vi "USB6343_Control_v1.6.2.vi"(8 "error in":errorcluster caption="错误输出", 10 "interface":T2, 11 "tasks":T3) -> ()   [LabVIEW 2013]
uses:
  <vilib>/DAQmx/read.llb/DAQmx Read (Analog 1D DBL NChan 1Samp).vi
  <vilib>/DAQmx/read.llb/DAQmx Read (Digital 1D Bool NChan 1Samp 1Line).vi
  <vilib>/DAQmx/read.llb/DAQmx Read (Counter DBL 1Chan 1Samp).vi
  <vilib>/DAQmx/write.llb/DAQmx Write (Digital 1D Bool NChan 1Samp 1Line).vi
  <vilib>/DAQmx/write.llb/DAQmx Write (Analog 1D DBL NChan 1Samp).vi
  <vilib>/DAQmx/miscellaneous.llb/DAQmx Fill In Error Info.vi
  <vilib>/DAQmx/configure/timing.llb/DAQmx Timing (Implicit).vi
panel:
  in  "stop":bool=TRUE
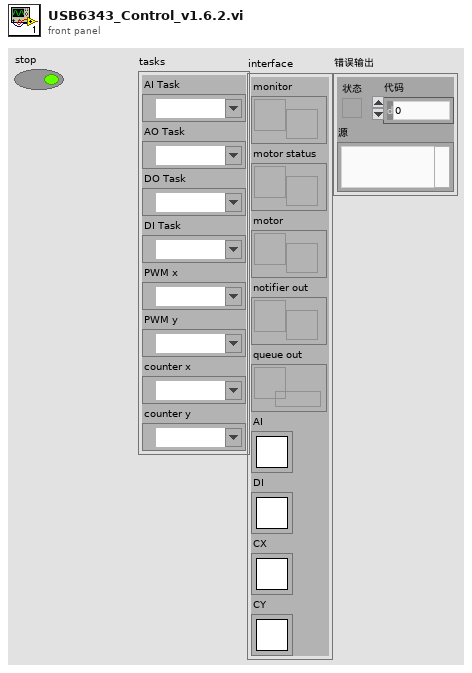
[diagram p1: front panel]
types:
  T1 = typedef "Semaphore RefNum" = refnum<k1>
  T2 = cluster{"monitor":refnum<user-event>, "motor status":refnum<user-event>, "motor":refnum<user-event>, "notifier out":refnum<notifier>, "queue out":refnum<queue>, "AI":T1, "DI":T1, "CX":T1, "CY":T1}
  T3 = cluster{"AI Task":refnum<k21>, "AO Task":refnum<k21>, "DO Task":refnum<k21>, "DI Task":refnum<k21>, "PWM x":refnum<k21>, "PWM y":refnum<k21>, "counter x":refnum<k21>, "counter y":refnum<k21>}
  T4 = cluster{"cmd":string, "channel":i32, "value":dbl, "on/off":bool, "return value":refnum<vi>}
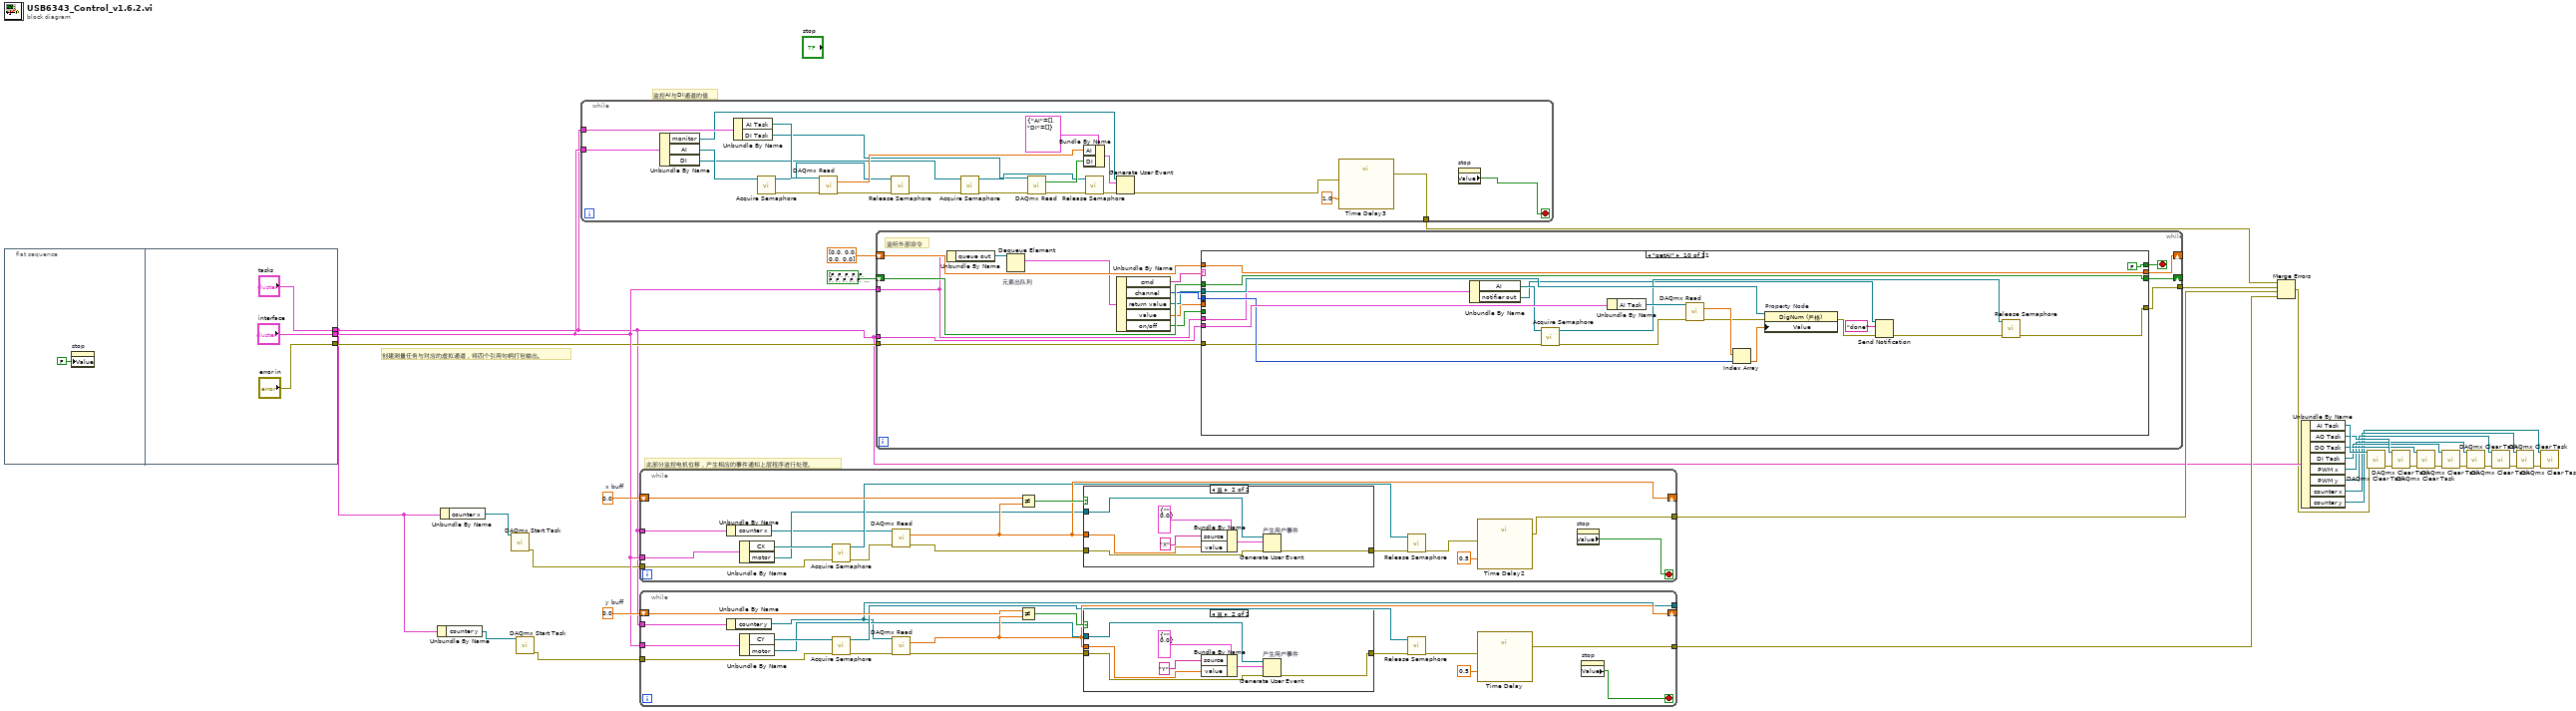
[diagram p0: block diagram]
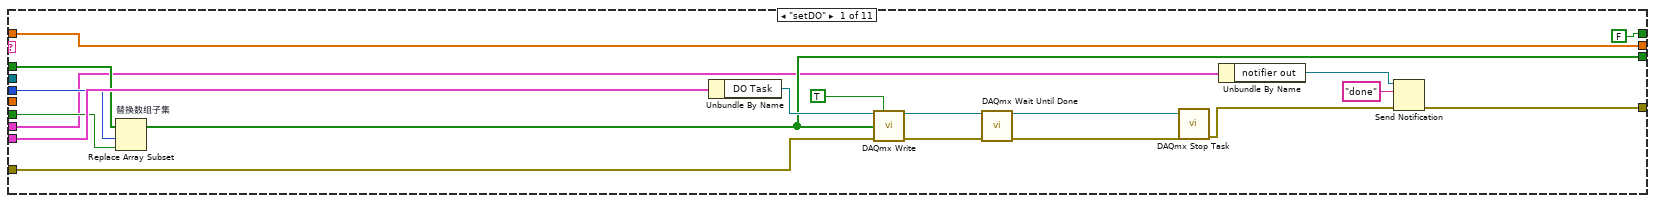
[diagram p4: hidden frame]
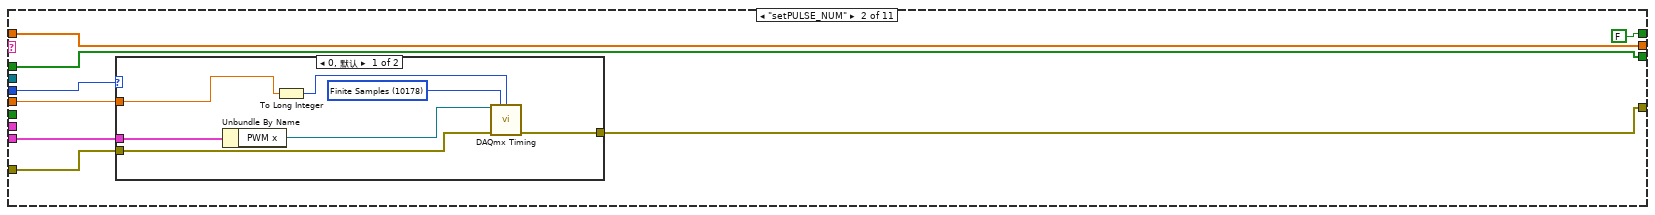
[diagram p5: hidden frame]
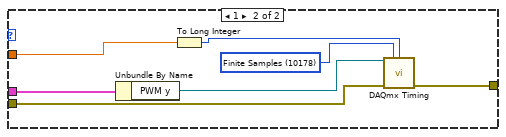
[diagram p6: hidden frame]
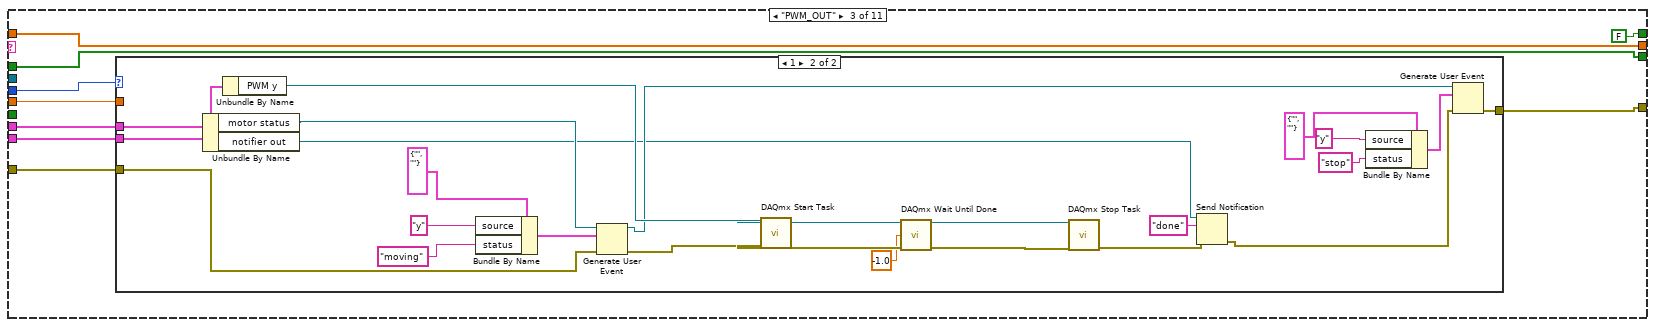
[diagram p7: hidden frame]
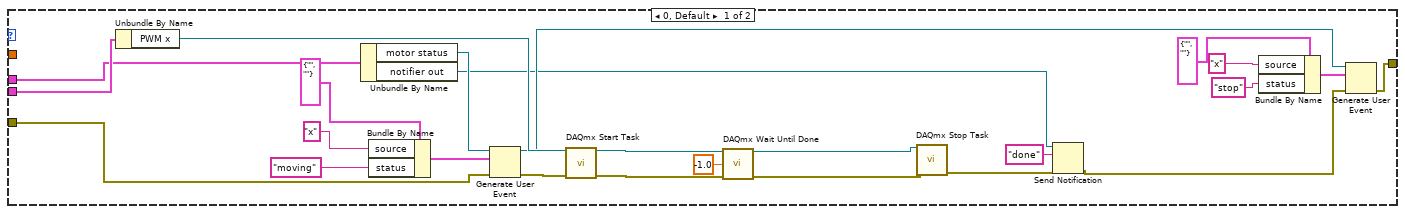
[diagram p8: hidden frame]
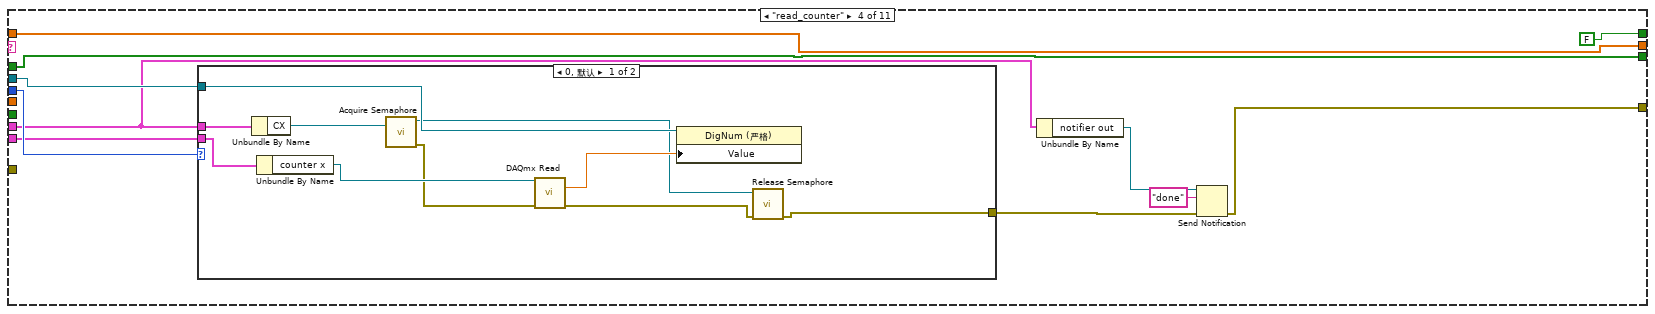
[diagram p9: hidden frame]
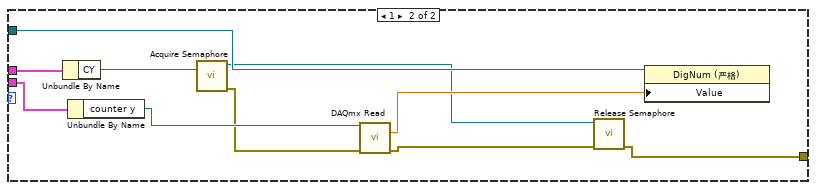
[diagram p10: hidden frame]
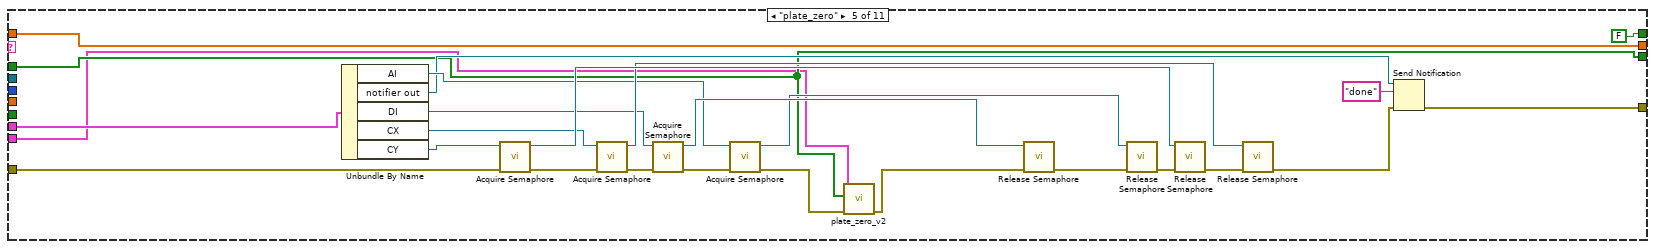
[diagram p11: hidden frame]
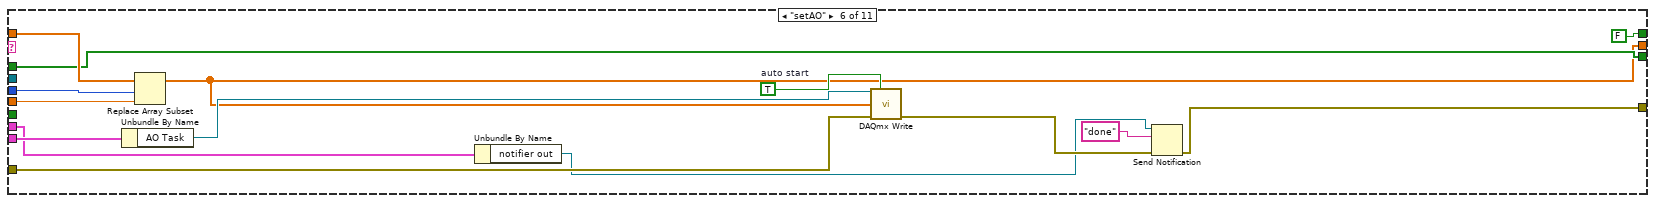
[diagram p12: hidden frame]
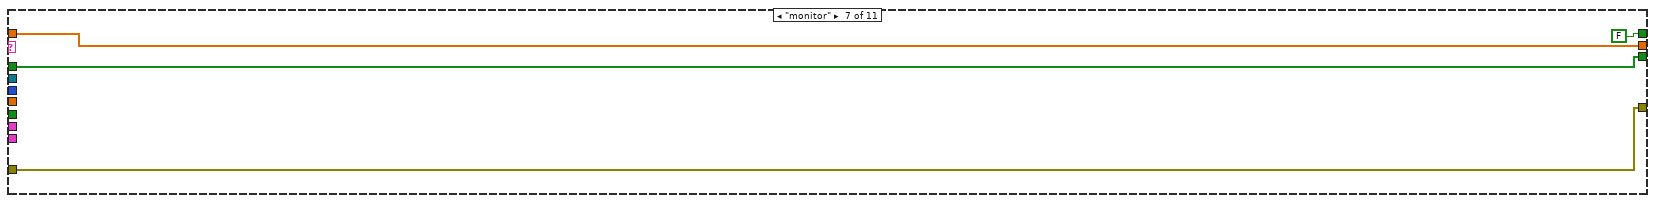
[diagram p13: hidden frame]
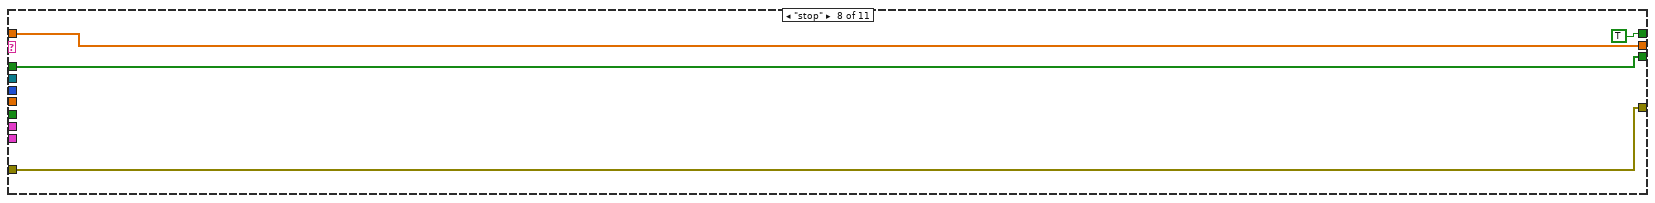
[diagram p14: hidden frame]
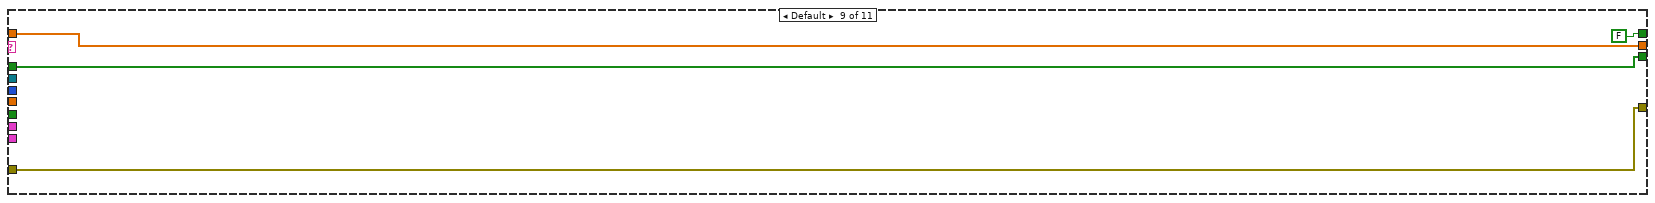
[diagram p15: hidden frame]
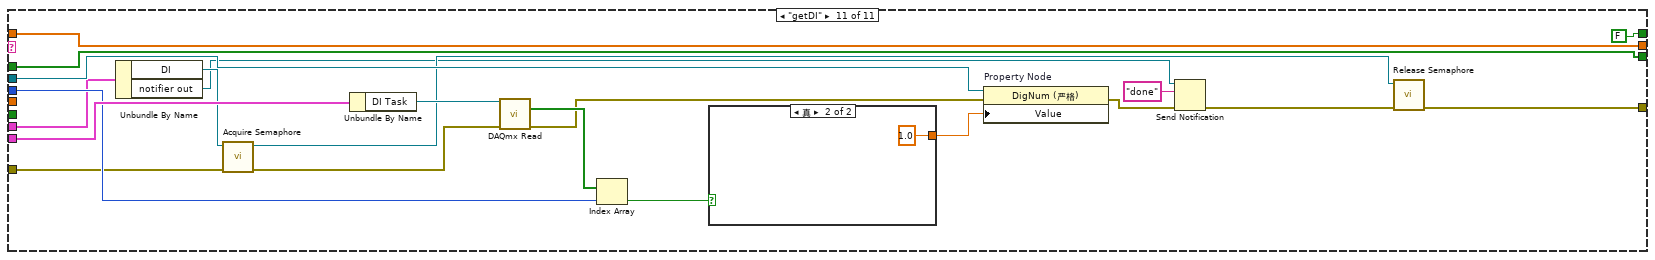
[diagram p16: hidden frame]
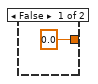
[diagram p17: hidden frame]
diagram:
  w28 = 0.0  # x buff
  w29 = 0.0  # y buff
  # "监控AI与DI通道的值"
  # "此部分监控电机位移，产生相应的事件通知上层程序进行处理。"
  # "创建测量任务与对应的虚拟通道，将四个引用句柄打包输出。"
  n1 = flat-sequence {
    tunnel: ["interface"] -> w27
    tunnel: ["error in"] -> w26
    tunnel: ["tasks"] -> w17
    frame #0 {
      n2 = property on="stop" class="Bool (严格)"("Value"=FALSE ("stop")) -> ()  [unwired: 2 in, 2 out]
    }
    frame #1 {
    }
  }
  n3 = Unbundle By Name(w17) -> ("counter y"=w22:refnum<k21>)
  n4 = Unbundle By Name(w17) -> ("counter x"=w23:refnum<k21>)
  n5 = call <vilib>:"DAQmx Start Task.vi"("task/channels in"=w23) -> ("error out"=w24:errorcluster)  [unwired: 13 in, 1 out]
  n6 = call <vilib>:"DAQmx Start Task.vi"("task/channels in"=w22) -> ("error out"=w25:errorcluster)  [unwired: 13 in, 1 out]
  n7 = while {
    tunnel: w17 -> [w57]
    tunnel: w27 -> [w42]
    tunnel: [w36] -> w21
    stop <- w37 stop-if-true
    n8 = Unbundle By Name(w42) -> ("monitor"=w41:refnum<user-event>, "AI"=w40:T1, "DI"=w39:T1)
    n9 = Unbundle By Name(w57) -> ("AI Task"=w58:refnum<k21>, "DI Task"=w38:refnum<k21>)
    n10 = call <vilib>:"Acquire Semaphore.vi"("semaphore"=w40) -> ("error out"=w43:errorcluster, "semaphore out"=w45:T1)  [unwired: 4 in, 1 out]
    n11 = call-poly <vilib>:"DAQmx Read.vi"("task/channels in"=w58, "error in"=w43) -> ("data"=w55:dbl[], "error out"=w50:errorcluster)  [unwired: 11 in, 1 out]
    n12 = call <vilib>:"Release Semaphore.vi"("error in (no error)"=w50, "semaphore"=w45) -> ("error out"=w49:errorcluster)  [unwired: 4 in, 1 out]
    n13 = call <vilib>:"Acquire Semaphore.vi"("error in (no error)"=w49, "semaphore"=w39) -> ("error out"=w48:errorcluster, "semaphore out"=w44:T1)  [unwired: 3 in, 1 out]
    n14 = call-poly <vilib>:"DAQmx Read.vi"("task/channels in"=w38, "error in"=w48) -> ("data"=w54:bool[], "error out"=w47:errorcluster)  [unwired: 11 in, 1 out]
    n15 = Bundle By Name(cluster=cluster{"AI":dbl[], "DI":bool[]} {"AI"=[], "DI"=[]} ("event data"), "AI"=w55, "DI"=w54) -> (w51:cluster{"AI":dbl[], "DI":bool[]})
    n16 = call <vilib>:"Release Semaphore.vi"("error in (no error)"=w47, "semaphore"=w44) -> ("error out"=w46:errorcluster)  [unwired: 4 in, 1 out]
    n17 = Generate User Event(user event=w41, event data cluster=w51, error in=w46) -> (error out=w53:errorcluster)  [unwired: 1 in, 1 out]
    n18 = call "Time Delay3"("error in (no error)"=w53, "Delay Time (s)"=1.0) -> ("error out"=w36:errorcluster)  [unwired: 9 in]
    n19 = property on="stop" class="Bool (严格)"() -> ("Value"=w37:bool)  [unwired: 2 in, 2 out]
  }
  n20 = while {
    shift-right: [w72] -> _
    shift-left: w28 -> [w75]
    tunnel: w27 -> [w66]
    tunnel: w17 -> [w63]
    tunnel: w24 -> [w61]
    tunnel: [w59] -> w19
    stop <- w60 stop-if-true
    n21 = Unbundle By Name(w63) -> ("counter x"=w62:refnum<k21>)
    n22 = Unbundle By Name(w66) -> ("CX"=w65:T1, "motor"=w64:refnum<user-event>)
    n23 = call <vilib>:"Acquire Semaphore.vi"("error in (no error)"=w61, "semaphore"=w65) -> ("error out"=w71:errorcluster, "semaphore out"=w68:T1)  [unwired: 3 in, 1 out]
    n24 = call-poly <vilib>:"DAQmx Read.vi"("task/channels in"=w62, "error in"=w71) -> ("data"=w72:dbl, "error out"=w73:errorcluster)  [unwired: 11 in, 1 out]
    n25 = Not Equal?(x=w75, y=w72) -> (x != y?=w74:bool)
    n26 = case shown="真" w74 {
      tunnel: w72 -> [_ w77]
      tunnel: w73 -> [w76 w80]
      tunnel: [w76 w79] -> w70
      tunnel: w64 -> [_ w78]
      frame False {
      }
      frame True {
        n27 = Bundle By Name(cluster=cluster{"source":string, "value":dbl} {"source"="", "value"=0.0} ("事件数据"), "source"="X", "value"=w77) -> (w81:cluster{"source":string, "value":dbl})
        n28 = Generate User Event "产生用户事件"(user event=w78, event data cluster=w81, error in=w80) -> (error out=w79:errorcluster)  [unwired: 1 in, 1 out]
      }
    }
    n29 = call <vilib>:"Release Semaphore.vi"("error in (no error)"=w70, "semaphore"=w68) -> ("error out"=w69:errorcluster)  [unwired: 4 in, 1 out]
    n30 = call "Time Delay2"("error in (no error)"=w69, "Delay Time (s)"=0.5) -> ("error out"=w59:errorcluster)  [unwired: 9 in]
    n31 = property on="stop" class="Bool (严格)"() -> ("Value"=w60:bool)  [unwired: 2 in, 2 out]
  }
  n32 = while {
    tunnel: [w87] -> _
    shift-right: [w97] -> _
    shift-left: w29 -> [w100]
    tunnel: w27 -> [w91]
    tunnel: w17 -> [w88]
    tunnel: w25 -> [w86]
    tunnel: [w84] -> w18
    stop <- w85 stop-if-true
    n33 = Unbundle By Name(w88) -> ("counter y"=w87:refnum<k21>)
    n34 = Unbundle By Name(w91) -> ("CY"=w90:T1, "motor"=w89:refnum<user-event>)
    n35 = call <vilib>:"Acquire Semaphore.vi"("error in (no error)"=w86, "semaphore"=w90) -> ("error out"=w96:errorcluster, "semaphore out"=w93:T1)  [unwired: 3 in, 1 out]
    n36 = call-poly <vilib>:"DAQmx Read.vi"("task/channels in"=w87, "error in"=w96) -> ("data"=w97:dbl, "error out"=w98:errorcluster)  [unwired: 11 in, 1 out]
    n37 = Not Equal?(x=w100, y=w97) -> (x != y?=w99:bool)
    n38 = case shown="真" w99 {
      tunnel: w97 -> [_ w102]
      tunnel: w98 -> [w101 w104]
      tunnel: [w101 w103] -> w95
      tunnel: w89 -> [_ w105]
      frame False {
      }
      frame True {
        n39 = Bundle By Name(cluster=cluster{"source":string, "value":dbl} {"source"="", "value"=0.0} ("事件数据"), "source"="Y", "value"=w102) -> (w106:cluster{"source":string, "value":dbl})
        n40 = Generate User Event "产生用户事件"(user event=w105, event data cluster=w106, error in=w104) -> (error out=w103:errorcluster)  [unwired: 1 in, 1 out]
      }
    }
    n41 = call <vilib>:"Release Semaphore.vi"("error in (no error)"=w95, "semaphore"=w93) -> ("error out"=w94:errorcluster)  [unwired: 4 in, 1 out]
    n42 = call "Time Delay"("error in (no error)"=w94, "Delay Time (s)"=0.5) -> ("error out"=w84:errorcluster)  [unwired: 9 in]
    n43 = property on="stop" class="Bool (严格)"() -> ("Value"=w85:bool)  [unwired: 2 in, 2 out]
  }
  n44 = while {
    tunnel: w17 -> [w118]
    tunnel: w26 -> [w124]
    shift-right: [w122] -> _
    shift-left: bool[] [FALSE, FALSE, FALSE, FALSE, FALSE, FALSE, FALSE, FALSE, FALSE, FALSE, FALSE, FALSE, FALSE, FALSE, FALSE, FALSE] -> [w123]
    shift-right: [w119] -> _
    shift-left: dbl[] [0.0, 0.0, 0.0, 0.0] ("data") -> [w120]
    tunnel: w27 -> [w111]
    tunnel: [w109] -> w20
    stop <- w121 stop-if-true
    # "监听外部命令"
    n45 = Unbundle By Name(w111) -> ("queue out"=w110:refnum<queue>)
    n46 = Dequeue Element "元素出队列"(queue=w110) -> (element=w117:T4)  [unwired: 2 in, 3 out]
    n47 = Unbundle By Name(w117) -> ("cmd"=w116:string, "channel"=w115:i32, "return value"=w114:refnum<vi>, "value"=w112:dbl, "on/off"=w113:bool)
    n48 = case shown="\"getAI\"" w116 {
      tunnel: w115 -> [w141 w145 w168 w235 _ w294 _ _ _ w324 w347]
      tunnel: w118 -> [w143 w148 w171 w234 w257 w296 _ _ _ w328 w349]
      tunnel: w124 -> [w135 w146 w169 _ w273 w289 w297 w301 w305 w317 w337]
      tunnel: w123 -> [w142 w149 w172 w225 w259 w292 w300 w304 w308 w322 w346]
      tunnel: w113 -> [w140 _ _ _ _ _ _ _ _ _ _]
      tunnel: [w133 w149 w172 w225 w259 w292 w300 w304 w308 w322 w346] -> w122
      tunnel: [FALSE FALSE FALSE FALSE FALSE FALSE FALSE TRUE FALSE FALSE FALSE] -> w121
      tunnel: w120 -> [w138 w150 w173 w226 w280 w293 w299 w302 w306 w321 w345]
      tunnel: [w138 w150 w173 w226 w280 w282 w299 w302 w306 w321 w345] -> w119
      tunnel: w114 -> [_ _ _ w233 _ _ _ _ _ w326 w348]
      tunnel: [w137 w144 w167 w228 w279 w286 w297 w301 w305 w313 w332] -> w109
      tunnel: w112 -> [_ w147 w170 _ _ w288 _ _ _ _ _]
      tunnel: w111 -> [w129 _ w166 w231 w265 w285 _ _ _ w311 w331]
      frame "setDO" {
        n49 = Replace Array Subset "替换数组子集"(array=w142, new element=w140, index=w141) -> (w133:bool[])
        n50 = Unbundle By Name(w143) -> ("DO Task"=w134:refnum<k21>)
        n51 = call-poly <vilib>:"DAQmx Write.vi"("task/channels in"=w134, "auto start"=TRUE, "data"=w133, "error in"=w135) -> ("task out"=w130:refnum<k21>, "error out"=w131:errorcluster)  [unwired: 9 in, 1 out]
        n52 = call <vilib>:"DAQmx Wait Until Done.vi"("task/channels in"=w130, "error in"=w131) -> ("task out"=w125:refnum<k21>, "error out"=w127:errorcluster)  [unwired: 12 in]
        n53 = call <vilib>:"DAQmx Stop Task.vi"("task/channels in"=w125, "error in"=w127) -> ("error out"=w126:errorcluster)  [unwired: 12 in, 1 out]
        n54 = Unbundle By Name(w129) -> ("notifier out"=w128:refnum<notifier>)
        n55 = Send Notification(notification="done" ("通知"), notifier=w128, error in (no error)=w126) -> (error out=w137:errorcluster)  [unwired: 1 out]
      }
      frame "setPULSE_NUM" {
        n56 = case shown="0, 默认" w145 {
          tunnel: w148 -> [w158 w165]
          tunnel: w147 -> [w153 w160]
          tunnel: w146 -> [w155 w162]
          tunnel: [w154 w161] -> w144
          frame 0, Default {
            w156 = 10178 items=["Finite Samples"=10178, "Continuous Samples"=10123, "Hardware Timed Single Point"=12522] ("sample mode")
            n57 = Unbundle By Name(w158) -> ("PWM x"=w157:refnum<k21>)
            n58 = To Long Integer(number=w153) -> (32bit integer=w152:i32)
            n59 = call-poly <vilib>:"DAQmx Timing.vi"("task/channels in"=w157, "sample mode"=w156, "samples per channel"=w152, "error in"=w155) -> ("error out"=w154:errorcluster)  [unwired: 10 in, 1 out]
          }
          frame 1 {
            w163 = 10178 items=["Finite Samples"=10178, "Continuous Samples"=10123, "Hardware Timed Single Point"=12522] ("sample mode")
            n60 = Unbundle By Name(w165) -> ("PWM y"=w164:refnum<k21>)
            n61 = To Long Integer(number=w160) -> (32bit integer=w159:i32)
            n62 = call-poly <vilib>:"DAQmx Timing.vi"("task/channels in"=w164, "sample mode"=w163, "samples per channel"=w159, "error in"=w162) -> ("error out"=w161:errorcluster)  [unwired: 10 in, 1 out]
          }
        }
      }
      frame "PWM_OUT" {
        n63 = case shown="1" w168 {
          tunnel: w171 -> [w199 w224]
          tunnel: w170 -> [_ _]
          tunnel: w169 -> [w191 w216]
          tunnel: [w184 w210] -> w167
          tunnel: w166 -> [w182 w207]
          frame 0, Default {
            n64 = Unbundle By Name(w199) -> ("PWM x"=w198:refnum<k21>)
            n65 = Unbundle By Name(w182) -> ("motor status"=w181:refnum<user-event>, "notifier out"=w176:refnum<notifier>)
            n66 = Bundle By Name(cluster=cluster{"source":string, " status":string} {"source"="", " status"=""} ("event data"), "source"="x", "status"="moving") -> (w189:cluster{"source":string, " status":string})
            n67 = Generate User Event(user event=w181, event data cluster=w189, error in=w191) -> (user event out=w183:refnum<user-event>, error out=w190:errorcluster)  [unwired: 1 in]
            n68 = call <vilib>:"DAQmx Start Task.vi"("task/channels in"=w198, "error in"=w190) -> ("task out"=w196:refnum<k21>, "error out"=w197:errorcluster)  [unwired: 12 in]
            n69 = call <vilib>:"DAQmx Wait Until Done.vi"("task/channels in"=w196, "timeout (sec)"=-1.0, "error in"=w197) -> ("task out"=w195:refnum<k21>, "error out"=w180:errorcluster)  [unwired: 11 in]
            n70 = call <vilib>:"DAQmx Stop Task.vi"("task/channels in"=w195, "error in"=w180) -> ("error out"=w179:errorcluster)  [unwired: 12 in, 1 out]
            n71 = Send Notification(notification="done", notifier=w176, error in (no error)=w179) -> (error out=w178:errorcluster)  [unwired: 1 out]
            n72 = Bundle By Name(cluster=cluster{"source":string, " status":string} {"source"="", " status"=""} ("event data"), "source"="x", "status"="stop") -> (w185:cluster{"source":string, " status":string})
            n73 = Generate User Event(user event=w183, event data cluster=w185, error in=w178) -> (error out=w184:errorcluster)  [unwired: 1 in, 1 out]
          }
          frame 1 {
            n74 = Unbundle By Name(w207) -> ("motor status"=w206:refnum<user-event>, "notifier out"=w201:refnum<notifier>)
            n75 = Unbundle By Name(w224) -> ("PWM y"=w223:refnum<k21>)
            n76 = Bundle By Name(cluster=cluster{"source":string, " status":string} {"source"="", " status"=""} ("event data"), "source"="y", "status"="moving") -> (w209:cluster{"source":string, " status":string})
            n77 = Generate User Event(user event=w206, event data cluster=w209, error in=w216) -> (user event out=w205:refnum<user-event>, error out=w215:errorcluster)  [unwired: 1 in]
            n78 = call <vilib>:"DAQmx Start Task.vi"("task/channels in"=w223, "error in"=w215) -> ("task out"=w221:refnum<k21>, "error out"=w222:errorcluster)  [unwired: 12 in]
            n79 = call <vilib>:"DAQmx Wait Until Done.vi"("task/channels in"=w221, "timeout (sec)"=-1.0, "error in"=w222) -> ("task out"=w219:refnum<k21>, "error out"=w220:errorcluster)  [unwired: 11 in]
            n80 = call <vilib>:"DAQmx Stop Task.vi"("task/channels in"=w219, "error in"=w220) -> ("error out"=w204:errorcluster)  [unwired: 12 in, 1 out]
            n81 = Send Notification(notification="done", notifier=w201, error in (no error)=w204) -> (error out=w203:errorcluster)  [unwired: 1 out]
            n82 = Bundle By Name(cluster=cluster{"source":string, " status":string} {"source"="", " status"=""} ("event data"), "source"="y", "status"="stop") -> (w211:cluster{"source":string, " status":string})
            n83 = Generate User Event(user event=w205, event data cluster=w211, error in=w203) -> (error out=w210:errorcluster)  [unwired: 1 in, 1 out]
          }
        }
      }
      frame "read_counter" {
        n84 = case shown="0, 默认" w235 {
          tunnel: w231 -> [w245 w255]
          tunnel: w234 -> [w243 w253]
          tunnel: w233 -> [w240 w250]
          tunnel: [w236 w246] -> w232
          frame 0, Default {
            n85 = Unbundle By Name(w245) -> ("CX"=w244:T1)
            n86 = Unbundle By Name(w243) -> ("counter x"=w242:refnum<k21>)
            n87 = call <vilib>:"Acquire Semaphore.vi"("semaphore"=w244) -> ("error out"=w241:errorcluster, "semaphore out"=w237:T1)  [unwired: 4 in, 1 out]
            n88 = call-poly <vilib>:"DAQmx Read.vi"("task/channels in"=w242, "error in"=w241) -> ("data"=w239:dbl, "error out"=w238:errorcluster)  [unwired: 11 in, 1 out]
            n89 = property class="DigNum (严格)"(reference=w240, "Value"=w239) -> ()  [unwired: 1 in, 2 out]
            n90 = call <vilib>:"Release Semaphore.vi"("error in (no error)"=w238, "semaphore"=w237) -> ("error out"=w236:errorcluster)  [unwired: 4 in, 1 out]
          }
          frame 1 {
            n91 = Unbundle By Name(w255) -> ("CY"=w254:T1)
            n92 = Unbundle By Name(w253) -> ("counter y"=w252:refnum<k21>)
            n93 = call <vilib>:"Acquire Semaphore.vi"("semaphore"=w254) -> ("error out"=w251:errorcluster, "semaphore out"=w247:T1)  [unwired: 4 in, 1 out]
            n94 = call-poly <vilib>:"DAQmx Read.vi"("task/channels in"=w252, "error in"=w251) -> ("data"=w249:dbl, "error out"=w248:errorcluster)  [unwired: 11 in, 1 out]
            n95 = call <vilib>:"Release Semaphore.vi"("error in (no error)"=w248, "semaphore"=w247) -> ("error out"=w246:errorcluster)  [unwired: 4 in, 1 out]
            n96 = property class="DigNum (严格)"(reference=w250, "Value"=w249) -> ()  [unwired: 1 in, 2 out]
          }
        }
        n97 = Unbundle By Name(w231) -> ("notifier out"=w230:refnum<notifier>)
        n98 = Send Notification(notification="done", notifier=w230, error in (no error)=w232) -> (error out=w228:errorcluster)  [unwired: 1 out]
      }
      frame "plate_zero" {
        n99 = Unbundle By Name(w265) -> ("AI"=w264:T1, "notifier out"=w260:refnum<notifier>, "DI"=w263:T1, "CX"=w262:T1, "CY"=w261:T1)
        n100 = call <vilib>:"Acquire Semaphore.vi"("error in (no error)"=w273, "semaphore"=w261) -> ("error out"=w275:errorcluster, "semaphore out"=w269:T1)  [unwired: 3 in, 1 out]
        n101 = call <vilib>:"Acquire Semaphore.vi"("error in (no error)"=w275, "semaphore"=w262) -> ("error out"=w274:errorcluster, "semaphore out"=w266:T1)  [unwired: 3 in, 1 out]
        n102 = call <vilib>:"Acquire Semaphore.vi"("error in (no error)"=w274, "semaphore"=w263) -> ("error out"=w277:errorcluster, "semaphore out"=w268:T1)  [unwired: 3 in, 1 out]
        n103 = call <vilib>:"Acquire Semaphore.vi"("error in (no error)"=w277, "semaphore"=w264) -> ("error out"=w258:errorcluster, "semaphore out"=w267:T1)  [unwired: 3 in, 1 out]
        n104 = call "plate_zero_v2.vi"("error in"=w258, "DO array"=w259, "tasks"=w257) -> ("error out"=w256:errorcluster)  [unwired: 8 in]
        n105 = call <vilib>:"Release Semaphore.vi"("error in (no error)"=w256, "semaphore"=w268) -> ("error out"=w276:errorcluster)  [unwired: 4 in, 1 out]
        n106 = call <vilib>:"Release Semaphore.vi"("error in (no error)"=w276, "semaphore"=w267) -> ("error out"=w272:errorcluster)  [unwired: 4 in, 1 out]
        n107 = call <vilib>:"Release Semaphore.vi"("error in (no error)"=w272, "semaphore"=w269) -> ("error out"=w271:errorcluster)  [unwired: 4 in, 1 out]
        n108 = call <vilib>:"Release Semaphore.vi"("error in (no error)"=w271, "semaphore"=w266) -> ("error out"=w270:errorcluster)  [unwired: 4 in, 1 out]
        n109 = Send Notification(notification="done", notifier=w260, error in (no error)=w270) -> (error out=w279:errorcluster)  [unwired: 1 out]
      }
      frame "setAO" {
        w291 = TRUE  # auto start
        n110 = Unbundle By Name(w296) -> ("AO Task"=w295:refnum<k21>)
        n111 = Replace Array Subset(array=w293, new element=w288, index=w294) -> (w282:dbl[])
        n112 = Unbundle By Name(w285) -> ("notifier out"=w284:refnum<notifier>)
        n113 = call-poly <vilib>:"DAQmx Write.vi"("task/channels in"=w295, "auto start"=w291, "data"=w282, "error in"=w289) -> ("error out"=w287:errorcluster)  [unwired: 9 in, 2 out]
        n114 = Send Notification(notification="done", notifier=w284, error in (no error)=w287) -> (error out=w286:errorcluster)  [unwired: 1 out]
      }
      frame "monitor" {
      }
      frame "stop" {
      }
      frame Default {
      }
      frame "getAI" {
        n115 = Unbundle By Name(w311) -> ("AI"=w310:T1, "notifier out"=w309:refnum<notifier>)
        n116 = call <vilib>:"Acquire Semaphore.vi"("error in (no error)"=w317, "semaphore"=w310) -> ("error out"=w316:errorcluster, "semaphore out"=w312:T1)  [unwired: 3 in, 1 out]
        n117 = Unbundle By Name(w328) -> ("AI Task"=w327:refnum<k21>)
        n118 = call-poly <vilib>:"DAQmx Read.vi"("task/channels in"=w327, "error in"=w316) -> ("data"=w325:dbl[], "error out"=w315:errorcluster)  [unwired: 11 in, 1 out]
        n119 = Index Array(array=w325, index=w324) -> (element=w323:dbl)
        n120 = property on="Property Node" class="DigNum (严格)"(reference=w326, error in=w315, "Value"=w323) -> (error out=w318:errorcluster)  [unwired: 1 out]
        n121 = Send Notification(notification="done" ("通知"), notifier=w309, error in (no error)=w318) -> (error out=w314:errorcluster)  [unwired: 1 out]
        n122 = call <vilib>:"Release Semaphore.vi"("error in (no error)"=w314, "semaphore"=w312) -> ("error out"=w313:errorcluster)  [unwired: 4 in, 1 out]
      }
      frame "getDI" {
        n123 = Unbundle By Name(w331) -> ("DI"=w330:T1, "notifier out"=w329:refnum<notifier>)
        n124 = call <vilib>:"Acquire Semaphore.vi"("error in (no error)"=w337, "semaphore"=w330) -> ("error out"=w336:errorcluster, "semaphore out"=w333:T1)  [unwired: 3 in, 1 out]
        n125 = Unbundle By Name(w349) -> ("DI Task"=w341:refnum<k21>)
        n126 = call-poly <vilib>:"DAQmx Read.vi"("task/channels in"=w341, "error in"=w336) -> ("data"=w340:bool[], "error out"=w335:errorcluster)  [unwired: 11 in, 1 out]
        n127 = Index Array "Index Array"(array=w340, index=w347) -> (element=w339:bool)
        n128 = case shown="真" w339 {
          tunnel: [0.0 1.0] -> w338
          frame False {
          }
          frame True {
          }
        }
        n129 = property on="Property Node" class="DigNum (严格)"(reference=w348, error in=w335, "Value"=w338) -> (error out=w342:errorcluster)  [unwired: 1 out]
        n130 = Send Notification(notification="done" ("通知"), notifier=w329, error in (no error)=w342) -> (error out=w334:errorcluster)  [unwired: 1 out]
        n131 = call <vilib>:"Release Semaphore.vi"("error in (no error)"=w334, "semaphore"=w333) -> ("error out"=w332:errorcluster)  [unwired: 4 in, 1 out]
      }
    }
  }
  n132 = Merge Errors(w21, w20, w19, w18) -> (w16:errorcluster)
  n133 = Unbundle By Name(w17) -> ("AI Task"=w15:refnum<k21>, "AO Task"=w14:refnum<k21>, "DO Task"=w13:refnum<k21>, "DI Task"=w12:refnum<k21>, "PWM x"=w11:refnum<k21>, "PWM y"=w10:refnum<k21>, "counter x"=w9:refnum<k21>, "counter y"=w8:refnum<k21>)
  n134 = call <vilib>:"DAQmx Clear Task.vi"("task in"=w15, "error in"=w16) -> ("error out"=w7:errorcluster)  [unwired: 13 in]
  n135 = call <vilib>:"DAQmx Clear Task.vi"("task in"=w14, "error in"=w7) -> ("error out"=w6:errorcluster)  [unwired: 13 in]
  n136 = call <vilib>:"DAQmx Clear Task.vi"("task in"=w13, "error in"=w6) -> ("error out"=w5:errorcluster)  [unwired: 13 in]
  n137 = call <vilib>:"DAQmx Clear Task.vi"("task in"=w12, "error in"=w5) -> ("error out"=w4:errorcluster)  [unwired: 13 in]
  n138 = call <vilib>:"DAQmx Clear Task.vi"("task in"=w11, "error in"=w4) -> ("error out"=w3:errorcluster)  [unwired: 13 in]
  n139 = call <vilib>:"DAQmx Clear Task.vi"("task in"=w10, "error in"=w3) -> ("error out"=w2:errorcluster)  [unwired: 13 in]
  n140 = call <vilib>:"DAQmx Clear Task.vi"("task in"=w9, "error in"=w2) -> ("error out"=w1:errorcluster)  [unwired: 13 in]
  n141 = call <vilib>:"DAQmx Clear Task.vi"("task in"=w8, "error in"=w1) -> ()  [unwired: 13 in, 1 out]
